vi "_048.vi"() -> ()   [LabVIEW 2024]
uses:
  <vilib>/Analysis/NI_AALBase.lvlib
panel:
  out "Min Time":u32
  out "Avg":dbl format="%0.2f"
  out "Max Time":u32
  out "o/p":dbl
  # "Measure Average Code Execution Time :"
  # "( Using LabVIEW )"
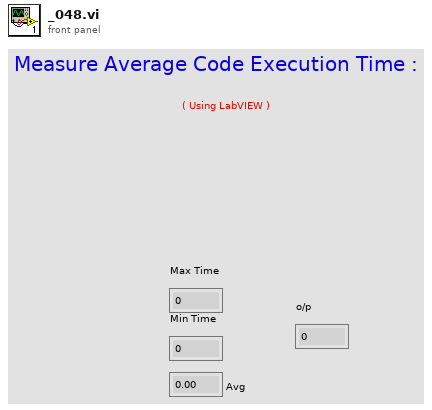
[diagram p1: front panel]
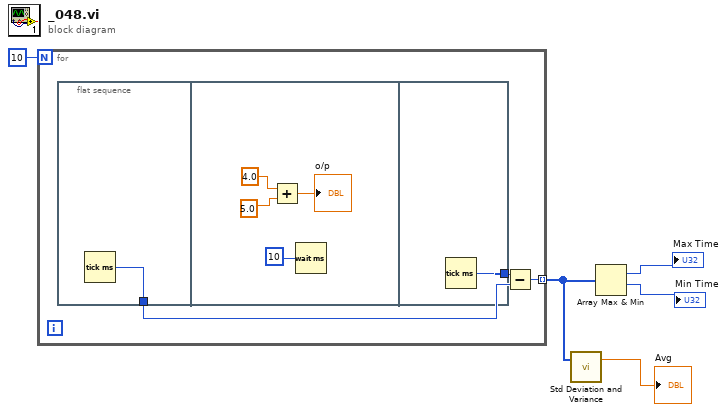
[diagram p0: block diagram]
diagram:
  n1 = for {
    N: 10 -> [_]
    tunnel: [w6] -> w3 mode=indexing
    n2 = flat-sequence {
      tunnel: [w9] -> w8
      tunnel: [w14] -> w7
      frame #0 {
        n3 = Tick Count (ms)() -> (millisecond timer value=w9:u32)
      }
      frame #1 {
        n4 = Add(x=4.0, y=5.0) -> (x+y=→"o/p":dbl)
        n5 = Wait (ms)(milliseconds to wait=u32 10 ("millisecond timer value")) -> ()  [unwired: 1 out]
      }
      frame #2 {
        n6 = Tick Count (ms)() -> (millisecond timer value=w14:u32)
      }
    }
    n7 = Subtract(x=w7, y=w8) -> (x-y=w6:u32)
  }
  n8 = call <vilib>:"Std Deviation and Variance.vi"("X"=w3) -> ("mean"=→"Avg":dbl)  [unwired: 1 in, 2 out]
  n9 = Array Max & Min(array=w3) -> (max value=→"Max Time":u32, min value=→"Min Time":u32)  [unwired: 2 out]
